vi "Download Package.vi"(8 "error in (no error)":errorcluster, 10 "URL":string, 11 "WebView2 Updater in":refnum<class "WebView2 Updater.lvclass">) -> (0 "error out":errorcluster, 3 "WebView2 Updater out":refnum<class "WebView2 Updater.lvclass">)   [LabVIEW 2020, in "WebView2 Updater.lvclass"]
uses:
  WebView2 Updater.lvclass
  WebView2 Updater.lvclass/WebView2 Updater.ctl
  <vilib>/httpClient/LabVIEWHTTPClient.lvlib
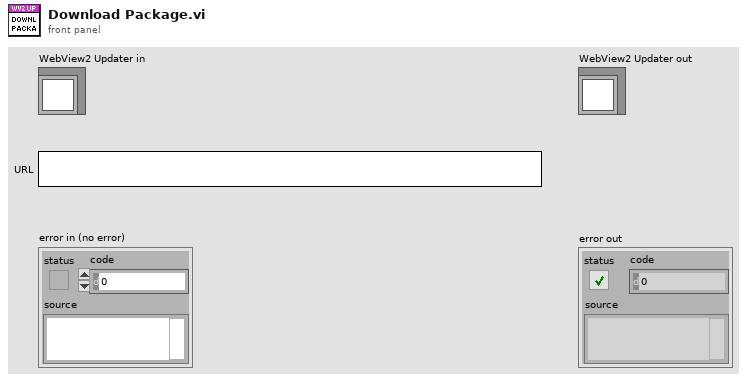
[diagram p1: front panel]
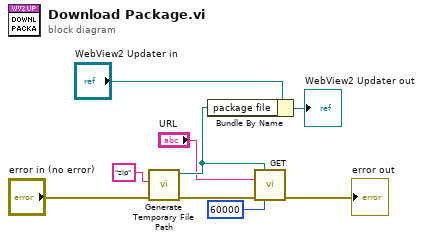
[diagram p0: block diagram]
diagram:
  n1 = call <vilib>:"Generate Temporary File Path.vi"("error in (no error)"="error in (no error)", "Temporary File Extension (tmp)"="zip") -> ("error out"=w5:errorcluster, "Unique Temporary File Path"=w8:path)  [unwired: 8 in]
  n2 = Bundle By Name(cluster="WebView2 Updater in", "package file"=w8) -> (→"WebView2 Updater out":refnum<class "WebView2 Updater.lvclass">)
  n3 = call <vilib>:"GET.vi"("output file"=w8, "url"="URL", "error in (no error)"=w5, "timeout (10000)"=60000) -> ("error out"=→"error out":errorcluster)  [unwired: 8 in, 3 out]
